vi "Report Humidity.vi"(8 "error in (no error)":errorcluster, 10 "Humidity":dbl, 11 "Device Manager in":refnum<class "Device Manager.lvclass">) -> (0 "error out":errorcluster, 3 "Device Manager out":refnum<class "Device Manager.lvclass">)   [LabVIEW 2020, in "Device Manager.lvlib" / "Device Manager.lvclass"]
uses:
  Device Manager.lvclass
  Device Manager.lvclass/Device Manager.ctl
  Panel/Panel Messages/Report Temperature Msg/Report Temperature Msg.lvclass/Report Temperature Msg.ctl
  <vilib>/ActorFramework/Message Enqueuer/Message Enqueuer.lvclass/Message Enqueuer.ctl
  Panel/Panel Messages/Report Temperature Msg/Report Temperature Msg.lvclass
  C:/Program Files/National Instruments/LabVIEW 2026/vi.lib/ActorFramework/Message/Message.lvclass
  Panel/Panel Messages/Report Humidity Msg/Report Humidity Msg.lvclass
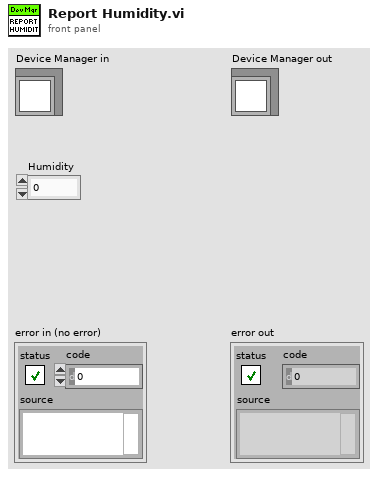
[diagram p1: front panel]
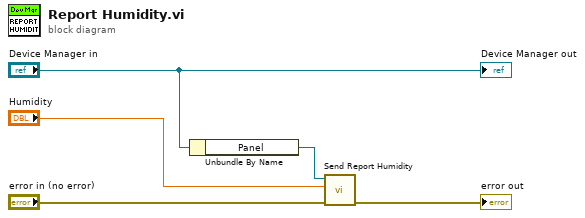
[diagram p0: block diagram]
diagram:
  n1 = Unbundle By Name("Device Manager in") -> ("Panel"=w5:refnum<class "Message Enqueuer.lvclass">)
  n2 = call "Send Report Humidity.vi"("error in (no error)"="error in (no error)", "Humidity"="Humidity", "Message Enqueuer"=w5) -> ("error out"=→"error out":errorcluster)  [unwired: 7 in, 1 out]
  "Device Manager out" <- "Device Manager in"
